vi "ABR-Analyze.vi"(0 "Runtime":T2, 7 "result":T1, 9 "Normalize individual?":bool, 11 "error in":errorcluster, 12 "Analysis in":T4, 13 "Graphs":T3) -> (4 "Runtime thru":T2, 6 "spread value":dbl, 14 "Analysis out":T4, 15 "error out":errorcluster)   [LabVIEW 2020]
uses:
  epl-vi-lib/Signal Synthesis VIs/4th Generation/Classes/SignalManager/SignalManager.lvclass
  Typedefs/ABR-Analysis State.ctl
  Threshold Estimation VIs/ABR3-Threshold Estimation Result.ctl
  Typedefs/ABR-Runtime Data.ctl
  Typedefs/ABR-Averaging Result.ctl
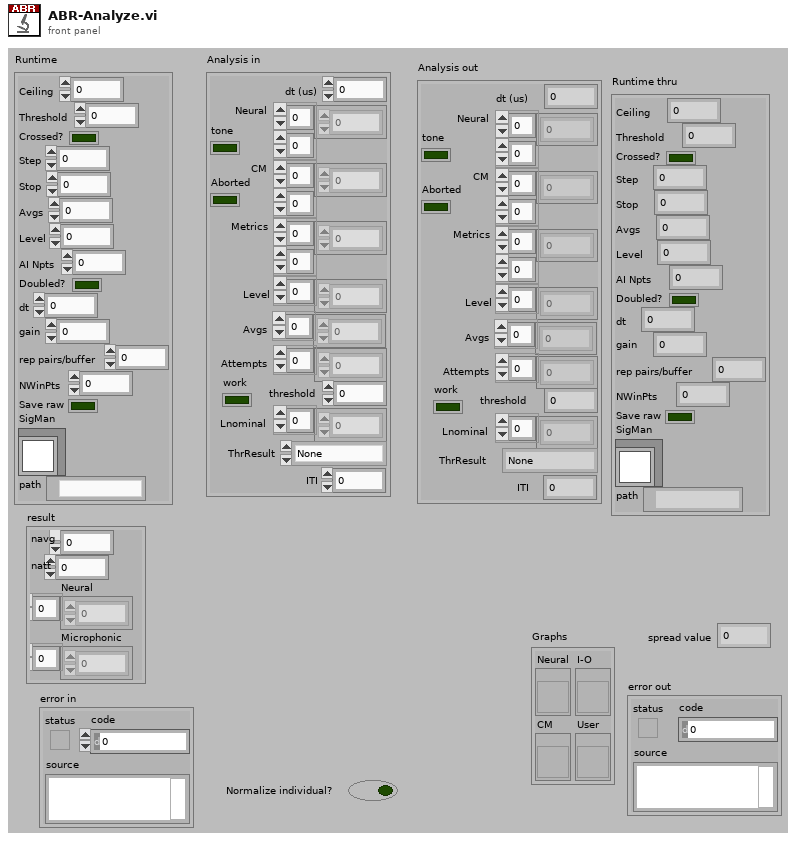
[diagram p1: front panel]
types:
  T1 = typedef "ABR-Averaging Result.ctl" = cluster{"navg":i32, "natt":i32, "Neural":dbl[], "Microphonic":dbl[]}
  T2 = typedef "ABR-Runtime Data.ctl" = cluster{"Ceiling":dbl, "Threshold":dbl, "Crossed?":bool, "Step":dbl, "Stop":i32, "Avgs":i32, "Level":dbl, "AI Npts":i32, "Doubled?":bool, "dt":dbl, "gain":dbl, "rep pairs/buffer":i32, "NWinPts":i32, "Save raw":bool, "SigMan":refnum<class "SignalManager.lvclass">, "path":path}
  T3 = cluster{"I-O":refnum<vi>, "Neural":refnum<vi>, "CM":refnum<vi>, "User":refnum<vi>}
  T4 = typedef "ABR-Analysis State.ctl" = cluster{"dt (us)":dbl, "Neural":dbl[][], "CM":dbl[][], "Metrics":dbl[][], "Level":dbl[], "Avgs":i32[], "Attempts":i32[], "Aborted":bool, "threshold":dbl, "Lnominal":dbl[], "tone":bool, "work":bool, "ThrResult":T5, "ITI":dbl}
  T5 = typedef "ABR3-Threshold Estimation Result.ctl" = enum16{"None", "Power", "Sigmoid", "Power (noisy)", "Suprathreshold", "Invalid"}
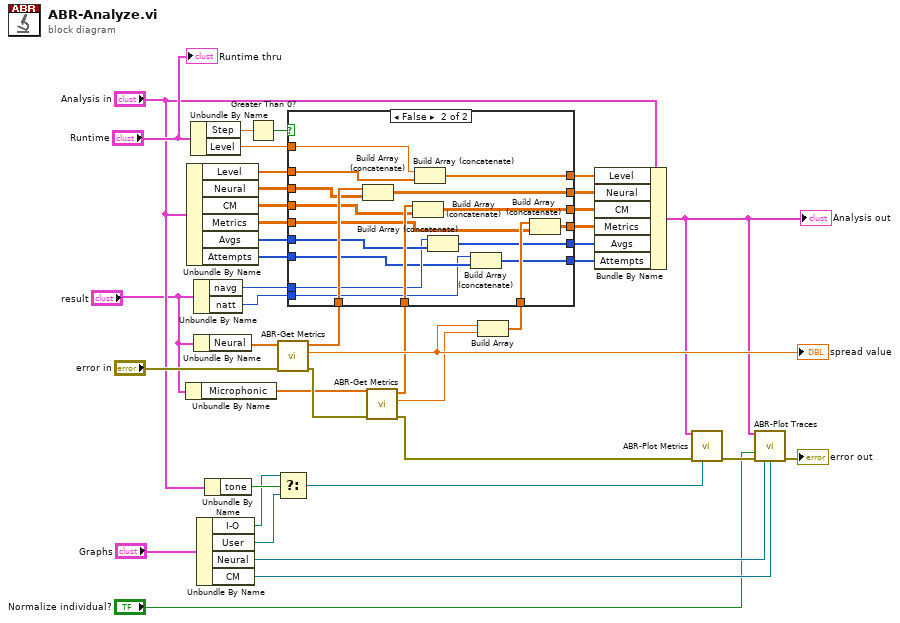
[diagram p0: block diagram]
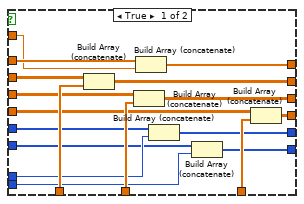
[diagram p2: hidden frame]
diagram:
  n1 = Unbundle By Name("result") -> ("Microphonic"=w1:dbl[])
  n2 = Unbundle By Name("Analysis in") -> ("Level"=w27:dbl[], "Neural"=w35:dbl[][], "CM"=w34:dbl[][], "Metrics"=w33:dbl[][], "Avgs"=w18:i32[], "Attempts"=w15:i32[])
  n3 = Unbundle By Name("Runtime") -> ("Step"=w5:dbl, "Level"=w25:dbl)
  n4 = Unbundle By Name("result") -> ("navg"=w17:i32, "natt"=w13:i32)
  n5 = Unbundle By Name("result") -> ("Neural"=w3:dbl[])
  n6 = Unbundle By Name("Graphs") -> ("I-O"=w8:refnum<vi>, "User"=w7:refnum<vi>, "Neural"=w21:refnum<vi>, "CM"=w20:refnum<vi>)
  n7 = Unbundle By Name("Analysis in") -> ("tone"=w9:bool)
  n8 = Greater Than 0?(x=w5) -> (x > 0?=w4:bool)
  n9 = call "ABR-Get Metrics.vi"("error in (no error)"="error in", "Data in"=w3) -> ("error out"=w29:errorcluster, "spread value"=w41:dbl, "Data out"=w39:dbl[])  [unwired: 7 in]
  "spread value" <- w41
  n10 = Select(t=w8, s=w9, f=w7) -> (s? t:f=w6:refnum<vi>)
  n11 = call "ABR-Get Metrics.vi"("error in (no error)"=w29, "Data in"=w1) -> ("error out"=w12:errorcluster, "spread value"=w37:dbl, "Data out"=w38:dbl[])  [unwired: 7 in]
  n12 = Build Array(w41, w37) -> (w40:dbl[])
  n13 = case shown="False" w4 {
    tunnel: w40 -> [w59 w77]
    tunnel: w39 -> [w58 w76]
    tunnel: w38 -> [w57 w75]
    tunnel: w35 -> [w56 w74]
    tunnel: w34 -> [w55 w73]
    tunnel: w33 -> [w54 w72]
    tunnel: [w53 w71] -> w32
    tunnel: [w52 w70] -> w31
    tunnel: [w51 w69] -> w30
    tunnel: w27 -> [w50 w68]
    tunnel: [w49 w67] -> w26
    tunnel: w25 -> [w48 w66]
    tunnel: w18 -> [w47 w65]
    tunnel: w17 -> [w46 w64]
    tunnel: [w45 w63] -> w16
    tunnel: w15 -> [w44 w62]
    tunnel: [w43 w61] -> w14
    tunnel: w13 -> [w42 w60]
    frame True {
      n14 = Build Array (concatenate)(w56, w58) -> (w53:dbl[][])
      n15 = Build Array (concatenate)(w55, w57) -> (w52:dbl[][])
      n16 = Build Array (concatenate)(w50, w48) -> (w49:dbl[])
      n17 = Build Array (concatenate)(w47, w46) -> (w45:i32[])
      n18 = Build Array (concatenate)(w44, w42) -> (w43:i32[])
      n19 = Build Array (concatenate)(w54, w59) -> (w51:dbl[][])
    }
    frame False {
      n20 = Build Array (concatenate)(w76, w74) -> (w71:dbl[][])
      n21 = Build Array (concatenate)(w75, w73) -> (w70:dbl[][])
      n22 = Build Array (concatenate)(w66, w68) -> (w67:dbl[])
      n23 = Build Array (concatenate)(w64, w65) -> (w63:i32[])
      n24 = Build Array (concatenate)(w60, w62) -> (w61:i32[])
      n25 = Build Array (concatenate)(w77, w72) -> (w69:dbl[][])
    }
  }
  n26 = Bundle By Name(cluster="Analysis in", "Level"=w26, "Neural"=w32, "CM"=w31, "Metrics"=w30, "Avgs"=w16, "Attempts"=w14) -> (w11:T4)
  "Analysis out" <- w11
  n27 = call "ABR-Plot Metrics.vi"("Analysis"=w11, "error in (no error)"=w12, "I-O"=w6) -> ("error out"=w23:errorcluster)  [unwired: 12 in]
  n28 = call "ABR-Plot Traces.vi"("Analysis"=w11, "Normalize individual?"="Normalize individual?", "error in (no error)"=w23, "Neural Ref"=w21, "CM Ref"=w20) -> ("error out"=→"error out":errorcluster)  [unwired: 10 in]
  "Runtime thru" <- "Runtime"
